vi "Test Read RS232.vi"() -> ()   [LabVIEW 2015]
uses:
  <vilib>/Instr/_visa.llb/VISA Configure Serial Port (Instr).vi
  <vilib>/Instr/_visa.llb/Select Event Type.ctl
panel:
  out "output array":string[](array[string])
  out "read buffer":string
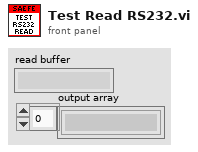
[diagram p1: front panel]
types:
  T1 = typedef "Select Event Type.ctl" = u32
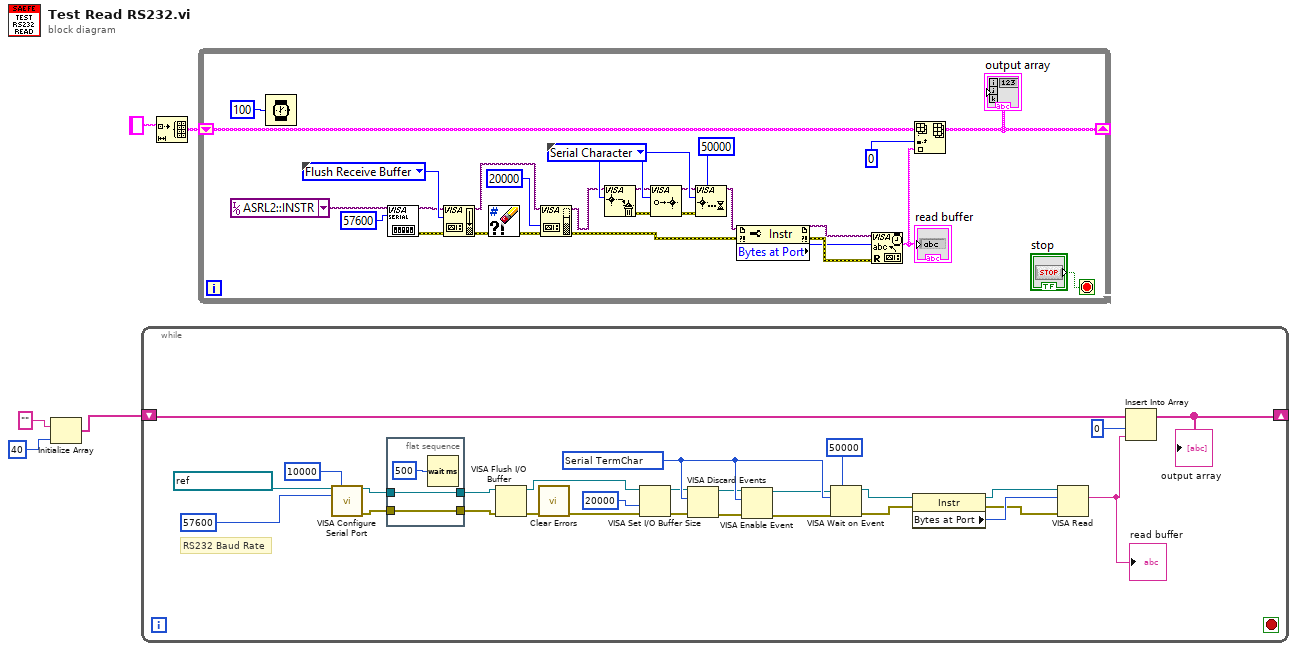
[diagram p0: block diagram]
diagram:
  n1 = Initialize Array("", 40 ("dimension size")) -> (w1:string[])
  n2 = while {
    shift-right: [w13] -> _
    shift-left: w1 -> [w12]
    stop <- _ stop-if-true
    w18 = T1 1073684516 items=["Service Request"=1073684491, "Trigger"=3221168138, "Clear"=1073684493, "VXI Signal"=1073684512, "VXI/VME Interrupt"=3221168161, "VXI/VME Sysfail"=1073684509, "VXI/VME Sysreset"=1073684510, "GPIB CIC"=1073684498, "GPIB Talk"=1073684499, "GPIB Listen"=1073684500, "PXI Interrupt"=1073684514, "Serial Break"=1073684515, "Serial TermChar"=1073684516, "Serial CTS"=1073684521, "Serial DSR"=1073684522, "Serial DCD"=1073684524, "Serial RI"=1073684526, "Serial Character"=1073684533, "USB Interrupt"=1073684535, "All Enabled"=1073709055] ("Event Type")
    # "RS232 Baud Rate"
    n3 = call-poly "VISA Configure Serial Port"("VISA resource name"=refnum<visa-resource-name> "ASRL2::INSTR", "timeout (10sec)"=u32 10000, "baud rate (9600)"=u32 57600 ("Baud Rate")) -> ("VISA resource name out"=w16:refnum<visa-resource-name>, "error out"=w14:errorcluster)  [unwired: 11 in]
    n4 = flat-sequence {
      tunnel: [w33] -> w17
      tunnel: w16 -> [w33]
      tunnel: [w32] -> w15
      tunnel: w14 -> [w32]
      frame #0 {
        n5 = Wait (ms)(milliseconds to wait=u32 500) -> ()  [unwired: 1 out]
      }
    }
    n6 = VISA Flush I/O Buffer(VISA resource name=w17, error in (no error)=w15) -> (VISA resource name out=w28:refnum<visa-resource-name>, error out=w27:errorcluster)  [unwired: 1 in]
    n7 = call <vilib>:"Clear Errors.vi"("error in (no error)"=w27) -> ("error out"=w26:errorcluster)  [unwired: 5 in, 1 out]
    n8 = VISA Set I/O Buffer Size(VISA resource name=w28, size (4096)=u32 20000, error in (no error)=w26) -> (VISA resource name out=w9:refnum<visa-resource-name>, error out=w5:errorcluster)  [unwired: 1 in]
    n9 = VISA Discard Events(8:w5, 10:w18, 11:w9) -> (0:w4:errorcluster, 3:w8:refnum<visa-resource-name>)  [unwired: 1 in]
    n10 = VISA Enable Event(8:w4, 10:w18, 11:w8) -> (0:w6:errorcluster, 3:w7:refnum<visa-resource-name>)  [unwired: 1 in]
    n11 = VISA Wait on Event(7:u32 50000 ("timeout (0)"), 8:w6, 10:w18, 11:w7) -> (0:w22:errorcluster, 3:w23:refnum<visa-resource-name>)  [unwired: 1 in, 2 out]
    n12 = property class="Instr"(reference=w23, error in=w22) -> (reference out=w20:refnum<visa-resource-name>, error out=w19:errorcluster, "Bytes at Port"=w21:u32)
    n13 = VISA Read(VISA resource name=w20, byte count=w21, error in (no error)=w19) -> (read buffer=w10:string)  [unwired: 3 out]
    "read buffer" <- w10
    n14 = Insert Into Array(array=w12, index=0, new element=w10) -> (w13:string[])
    "output array" <- w13
  }
